vi "Read Multiple Event Registration.vi"(6 "number of event structures":u16=2, 7 "subchannel (0)":i32, 10 "channel in":T1) -> (2 "event registration refnums":refnum<event-registration>[](array[refnum]))   [LabVIEW 2019, in "Event MessengerM.lvlib"]
doc: "Reads multiple refnums for an Event MessengerM channel and makes the refnums available to one or more Event structures.\n\nUnlike the reader endpoints of other channel templates, this reader endpoint must be placed outside the While Loop and can execute only once.\n\nUse one Event structure to handle events whenever possible. Use the Build Array or Bundle functions to combine multiple event registration refnums for a single Event structure.\n\nTo allow multiple Event structures to read event registration refnums from this endpoint, you must use the Index Array function to index the event registration refnums and wire each refnum to the dynamic event terminal of each Event structure so that each Event structure receives its own copy of the events from the channel.\n\nDo not fork the event registration refnums to multiple Event structures. Doing so creates undefined behavior that may result in race conditions or deadlocks in your application."
uses:
  Event MessengerM.lvlib
  ChannelOp.ctl
  ))Channel.ctl
  Event Data.ctl
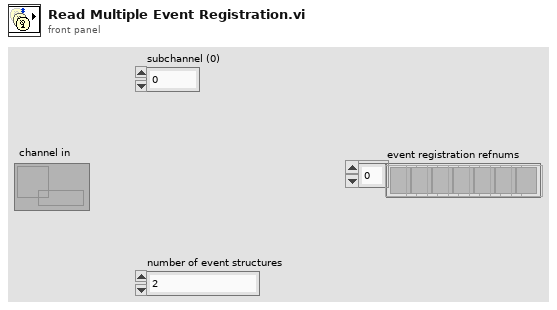
[diagram p1: front panel]
types:
  T1 = typedef "Event MessengerM.lvlib/))Channel.ctl" = refnum<queue>
  T2 = typedef "Event MessengerM.lvlib/ChannelOp.ctl" = enum16{"init", "write", "register", "replicate", "probe"}
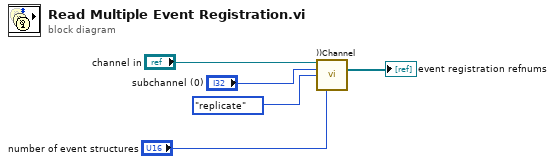
[diagram p0: block diagram]
diagram:
  n1 = call "))Channel.vi"("channel in"="channel in", "subchannel"="subchannel (0)", "channelOp"=ChannelOp."replicate", "# event structures"="number of event structures") -> ("event registration refnums"=→"event registration refnums":refnum<event-registration>[])  [unwired: 7 in, 4 out]
